vi "Doc_Builder_Write_Header.vi"(9 "Prefix String":string, 10 "Item Name":string, 11 "NI_report in":refnum<class "NI_report.lvclass">) -> (3 "NI_report out":refnum<class "NI_report.lvclass">)   [LabVIEW 2019]
uses:
  <vilib>/Utility/NIReport.llb/NI_report.lvclass
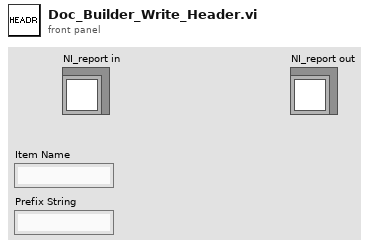
[diagram p1: front panel]
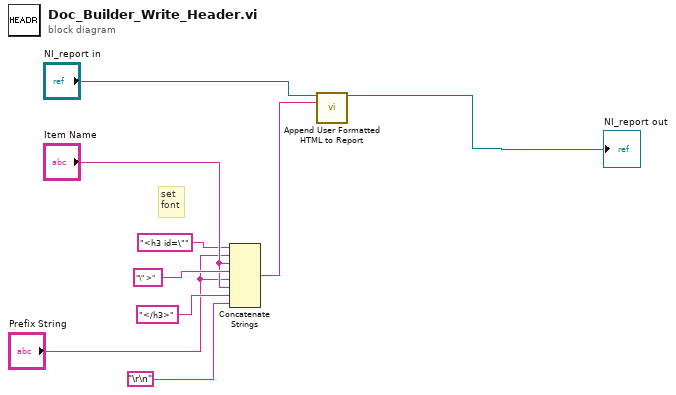
[diagram p0: block diagram]
diagram:
  # "set \nfont"
  n1 = Concatenate Strings("<h3 id=\"" ("text"), "Prefix String", "Item Name", "\" >" ("string"), "Prefix String", "Item Name", "</h3>" ("text"), "\r\n") -> (w1:string)
  n2 = call-dynamic "Append User Formatted HTML to Report.vi"("report in"="NI_report in", "HTML text"=w1) -> ("report out"=→"NI_report out":refnum<class "NI_report.lvclass">)  [unwired: 12 in, 1 out]
